vi "Control refrence holder.vi"(1 "Action(GET)":enum16{"GET", "SET"}(ring), 5 "Controll collection":T1, 7 "Controlls in":refnum<vi>[](array[refnum]), 11 "error in (no error)":errorcluster) -> (8 "Controlls out":refnum<vi>[](array[refnum]), 15 "error out":errorcluster)   [LabVIEW 2011]
uses:
  Controll refrence groups.ctl
  <vilib>/Utility/VariantDataType/GetNumericInfo.vi
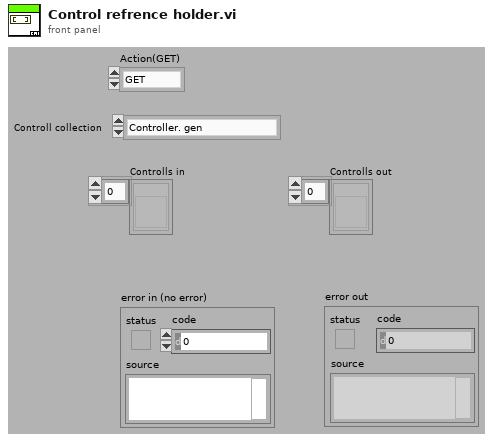
[diagram p1: front panel]
types:
  T1 = typedef "Controll refrence groups.ctl" = enum16{"Controller. gen", "Controller . High G", "Stroker", "PCP Online", "PCP Local", "PCP HV On", "Driller", "Stroker Cmd Buttons", "Stroker Anchor Cmd Buttons", "Controller Relay Buttons", "PCP Start Telemetry", "PCP Start Motor", "Tractor", "Modem Status"}
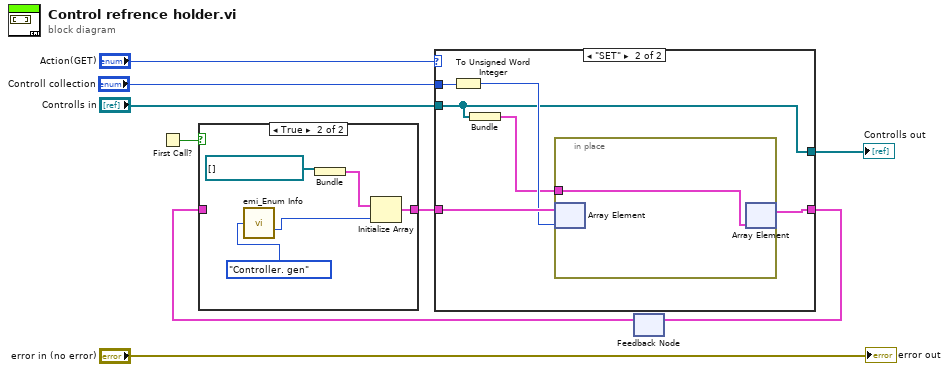
[diagram p0: block diagram]
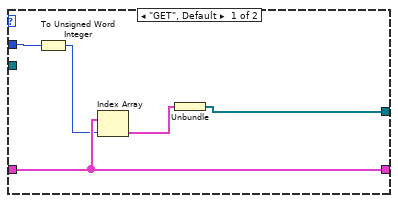
[diagram p3: hidden frame]
diagram:
  n1 = First Call?() -> (First Call?: T/F=w6:bool)
  n2 = feedback #1() -> (w7:cluster{"Controlls":refnum<vi>[]}[])  [unwired: 1 in]
  n3 = case shown="True" w6 {
    tunnel: w7 -> [w10 _]
    tunnel: [w10 w15] -> w4
    frame False {
    }
    frame True {
      n4 = call "emi_Enum Info.vi"("Enum"=Controll_refrence_groups."Controller. gen" ("Controll collection")) -> ("Numb Elements"=w13:i32)  [unwired: 11 in, 3 out]
      n5 = Bundle("Controlls"=refnum<vi>[] []) -> (w11:cluster{"Controlls":refnum<vi>[]})  [unwired: 1 in]
      n6 = Initialize Array(w11, w13) -> (w15:cluster{"Controlls":refnum<vi>[]}[])
    }
  }
  n7 = case shown="\"SET\"" "Action(GET)" {
    tunnel: [w20 w23] -> w5
    tunnel: w4 -> [w20 w25]
    tunnel: "Controlls in" -> [_ w21]
    tunnel: "Controll collection" -> [w19 w26]
    tunnel: [w16 w21] -> w1
    frame "GET", Default {
      n8 = To Unsigned Word Integer(number=w19) -> (unsigned 16bit integer=w18:u16)
      n9 = Index Array(array=w20, index=w18) -> (element=w17:cluster{"Controlls":refnum<vi>[]})
      n10 = Unbundle(w17) -> ("Controlls"=w16:refnum<vi>[])
    }
    frame "SET" {
      n11 = To Unsigned Word Integer(number=w26) -> (unsigned 16bit integer=w24:u16)
      n12 = Bundle("Controlls in"=w21) -> (w22:cluster{"Controlls in":refnum<vi>[]})  [unwired: 1 in]
      n13 = in-place {
        in-place-border: w22 -> [w27]
        n14 = in-place-array #2(w25, w24) -> ()  [unwired: 1 out]
        n15 = in-place-array #2(w27) -> (w23:cluster{"Controlls":refnum<vi>[]}[])  [unwired: 1 out]
      }
    }
  }
  "Controlls out" <- w1
  n16 = feedback-in #1(w5) -> ()
  "error out" <- "error in (no error)"
